vi "INI Extensions Global.vi"() -> ()   [LabVIEW 2011]
uses:
  Type Defs/INI Extensions Cluster.ctl
panel:
  in  "INI Extensions":T1={"Type Descriptions Path"=path "Inifile Extensions/TypeDescriptions.ini", "Pre-Defined Type Names"=[], "Pre-Defined Type Info"=[], "Text Lists"=[]}
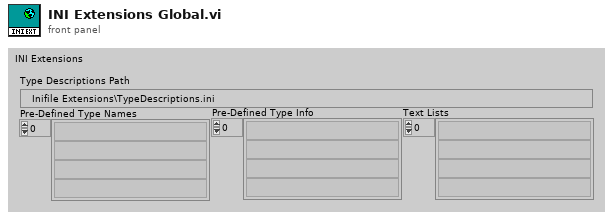
[diagram p1: front panel]
types:
  T1 = typedef "INI Extensions Cluster.ctl" = cluster{"Type Descriptions Path":path, "Pre-Defined Type Names":string[], "Pre-Defined Type Info":string[], "Text Lists":string[]}
diagram:
